vi "000 Data Edit Panel.vi"() -> (2 "OK?":bool)   [LabVIEW 2020]
panel:
  in  "Cancle":bool
  in  "OK":bool
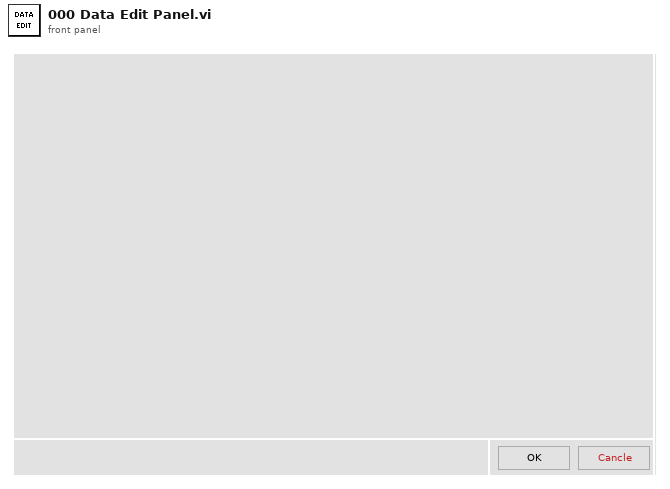
[diagram p1: front panel]
types:
  T1 = cluster{"UI":refnum<queue>, "UE":refnum<user-event>}
  T2 = cluster{"Queue":cluster{"UI":refnum<queue>, "UE":refnum<user-event>}, "OK?":bool}
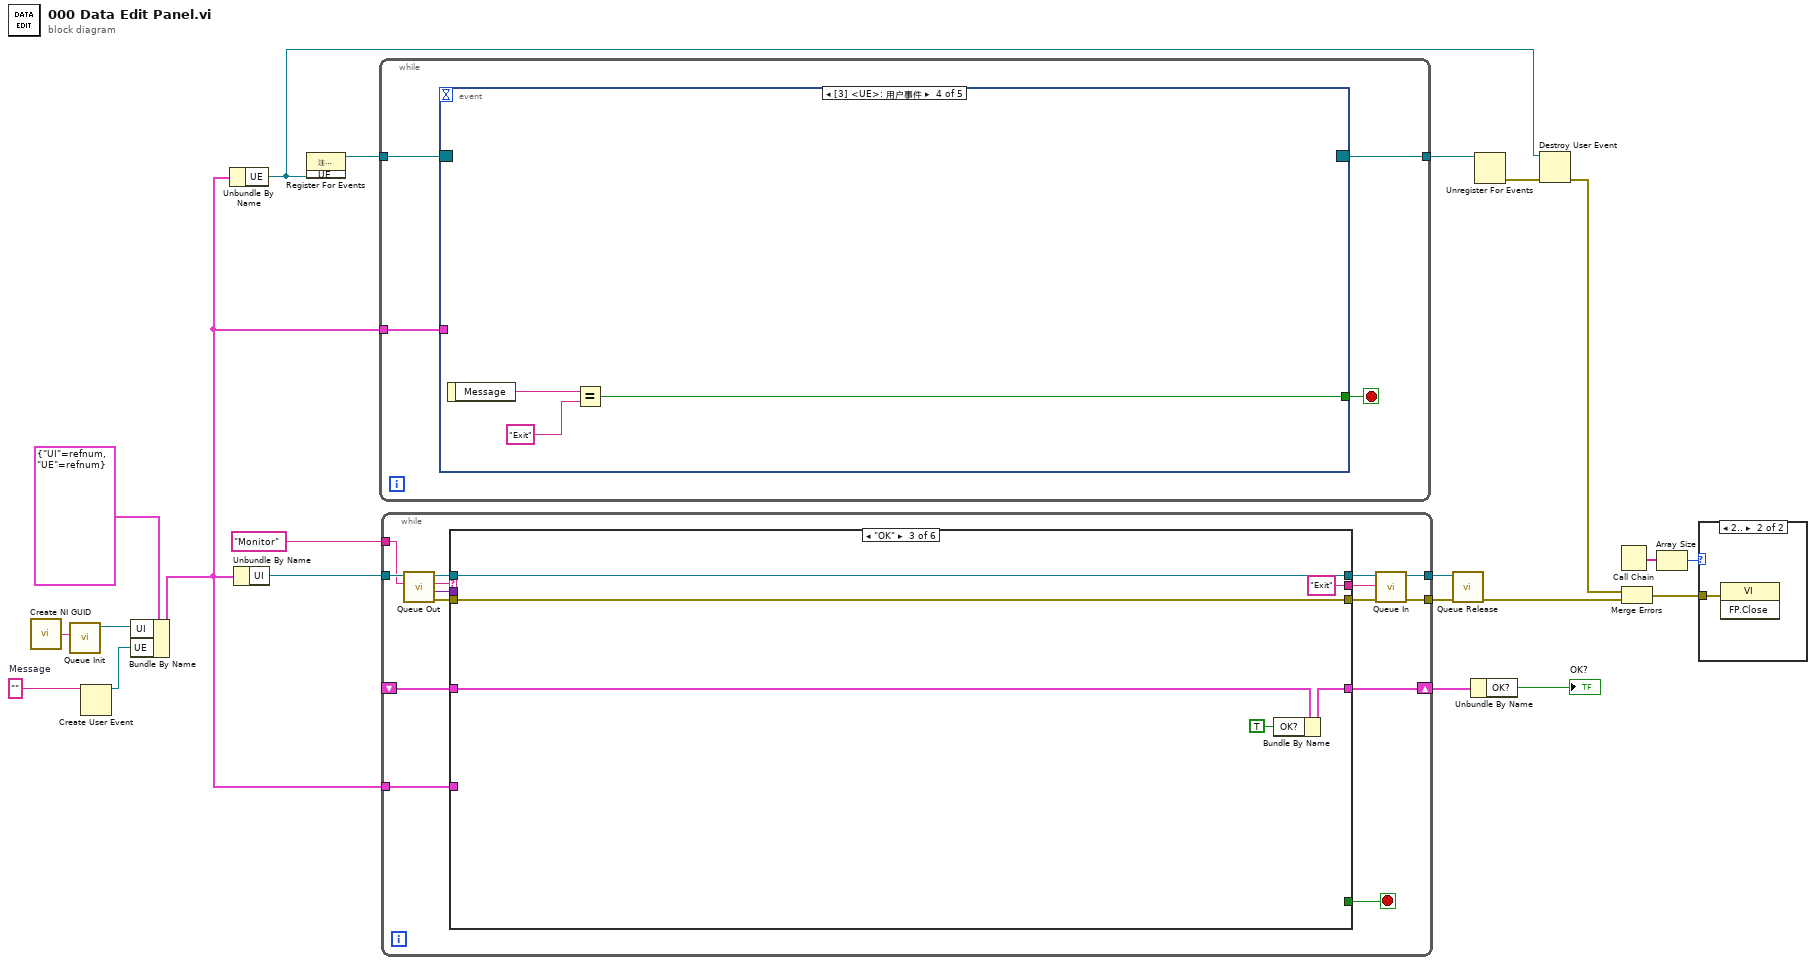
[diagram p0: block diagram]
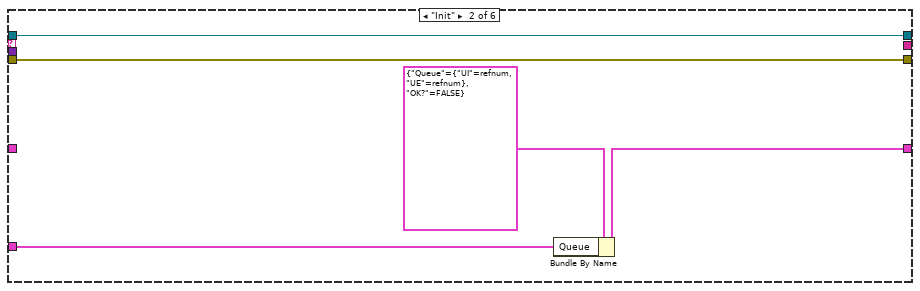
[diagram p4: hidden frame]
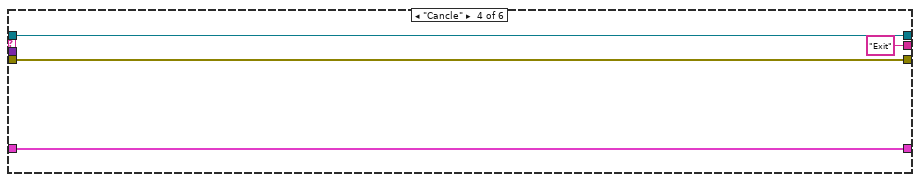
[diagram p5: hidden frame]
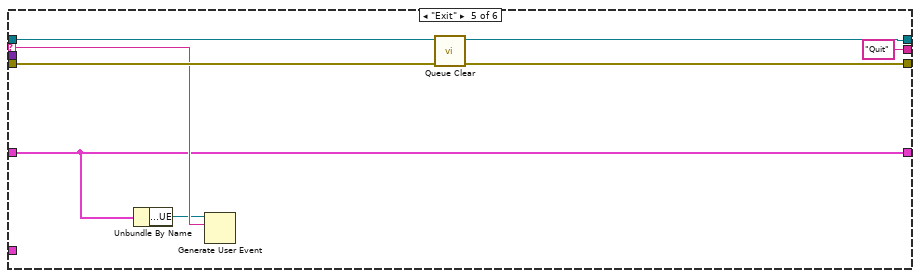
[diagram p6: hidden frame]
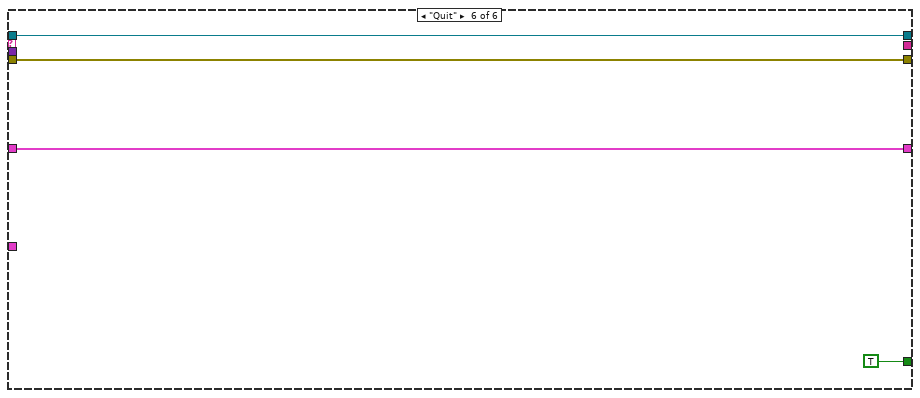
[diagram p7: hidden frame]
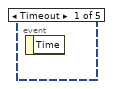
[diagram p8: hidden frame]
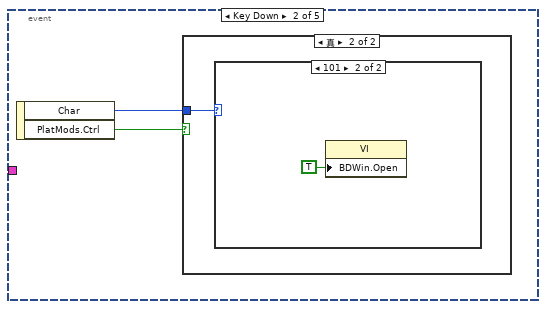
[diagram p9: hidden frame]
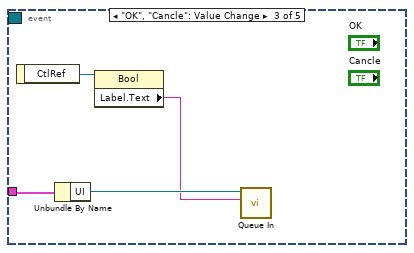
[diagram p12: hidden frame]
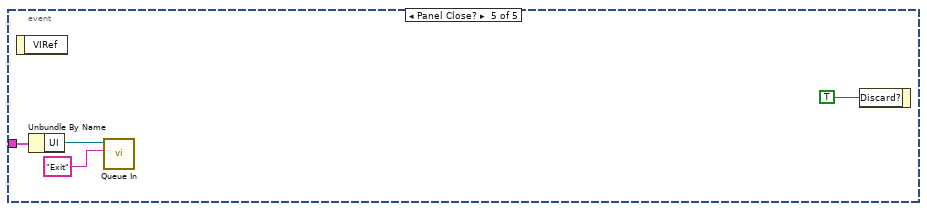
[diagram p13: hidden frame]
diagram:
  w10 = ""  # Message
  n1 = call <vilib>:"Create NI GUID.vi"() -> ("NI GUID"=w8:string)
  n2 = call "Queue Init.vi"("Queue Name"=w8) -> ("Queue Out"=w7:refnum<queue>)  [unwired: 8 in, 2 out]
  n3 = Create User Event(user event datatype=w10) -> (user event=w6:refnum<user-event>)  [unwired: 1 in, 1 out]
  n4 = Bundle By Name(cluster=T1 {"UI"=refnum, "UE"=refnum} ("Queue Ref Out"), "UI"=w7, "UE"=w6) -> (w5:T1)
  n5 = Unbundle By Name(w5) -> ("UE"=w4:refnum<user-event>)
  n6 = Unbundle By Name(w5) -> ("UI"=w16:refnum<queue>)
  n7 = register-events(w4) -> (reference out=w11:refnum<event-registration>)  [unwired: 2 in, 1 out]
  n8 = while {
    tunnel: w11 -> [w25]
    tunnel: [w23] -> w12
    tunnel: w5 -> [w22]
    stop <- w24 stop-if-true
    n9 = event shown="[3] <UE>: 用户事件" {
      selector: w25 -> [_ _ _ _ _]
      dyn-events: [_ _ _ _ _] -> w23
      timeout: _ -> [_ _ _ _ _]
      tunnel: [_ _ _ w34 _] -> w24
      tunnel: w22 -> [_ _ w33 _ w39]
      event Timeout {
        n10 = event-data() -> ()  [unwired: 1 in, 1 out]
      }
      event Key Down {
        n11 = event-data() -> ("Char"=w27:i16, "PlatMods.Ctrl"=w26:bool)  [unwired: 1 in]
        n12 = case shown="真" w26 {
          tunnel: w27 -> [_ w28]
          frame False {
          }
          frame True {
            n13 = case shown="101" w28 {
              frame 0, Default {
              }
              frame 101 {
                n14 = property class="VI"("BDWin.Open"=TRUE ("程序框图窗口:打开")) -> ()  [unwired: 2 in, 2 out]
              }
            }
          }
        }
      }
      event "OK", "Cancle": Value Change {
        n15 = event-data() -> ("CtlRef"=w31:refnum<vi>)  [unwired: 1 in]
        n16 = Unbundle By Name(w33) -> ("UI"=w32:refnum<queue>)
        n17 = property class="Bool"(reference=w31) -> ("Label.Text"=w30:string)  [unwired: 1 in, 2 out]
        n18 = call "Queue In.vi"("Message"=w30, "Queue In"=w32) -> ()  [unwired: 8 in, 2 out]
      }
      event User Event {
        n19 = event-data() -> ("Message"=w36:string)  [unwired: 1 in]
        n20 = Equal?(x=w36, y="Exit") -> (x = y?=w34:bool)
      }
      event Panel Close? {
        n21 = event-data() -> ()  [unwired: 1 in, 1 out]
        n22 = Unbundle By Name(w39) -> ("UI"=w38:refnum<queue>)
        n23 = call "Queue In.vi"("Message"="Exit", "Queue In"=w38) -> ()  [unwired: 8 in, 2 out]
        n24 = event-data("Discard?"=TRUE ("放弃？")) -> ()  [unwired: 1 in, 1 out]
      }
    }
  }
  n25 = while {
    tunnel: w16 -> [w51]
    tunnel: [w48] -> w14
    tunnel: [w47] -> w15
    tunnel: w5 -> [w44]
    shift-right: [w43] -> w3
    shift-left: _ -> [w42]
    tunnel: "Monitor" ("Monitor") -> [w41]
    stop <- w55 stop-if-true
    n26 = call "Queue Out.vi"("Monitor"=w41, "Queue In"=w51) -> ("error out"=w54:errorcluster, "Data"=w52:variant, "Message"=w53:string, "Queue Out"=w50:refnum<queue>)  [unwired: 5 in, 1 out]
    n27 = case shown="\"OK\"" w53 {
      selector: w53 -> [_ _ _ _ w76 _]
      tunnel: w50 -> [w58 w63 w69 w73 w80 w84]
      tunnel: w54 -> [w57 w62 w68 w72 w78 w85]
      tunnel: [w58 w63 w69 w73 w79 w84] -> w49
      tunnel: [w57 w62 w68 w72 w77 w85] -> w46
      tunnel: [_ _ "Exit" "Exit" "Quit" _] -> w45
      tunnel: [_ _ _ _ _ TRUE] -> w55
      tunnel: w52 -> [_ _ _ _ _ _]
      tunnel: w44 -> [_ w59 _ _ _ _]
      tunnel: [w56 w60 w66 w71 w74 w82] -> w43
      tunnel: w42 -> [w56 _ w67 w71 w74 w82]
      frame "eee", Default {
      }
      frame "Init" {
        n28 = Bundle By Name(cluster=T2 {"Queue"={"UI"=refnum, "UE"=refnum}, "OK?"=FALSE}, "Queue"=w59) -> (w60:T2)
      }
      frame "OK" {
        n29 = Bundle By Name(cluster=w67, "OK?"=TRUE) -> (w66:T2)
      }
      frame "Cancle" {
      }
      frame "Exit" {
        n30 = Unbundle By Name(w74) -> ("Queue.UE"=w75:refnum<user-event>)
        n31 = Generate User Event(user event=w75, event data cluster=w76) -> ()  [unwired: 2 in, 2 out]
        n32 = call "Queue Clear.vi"("error in (no error)"=w78, "Queue In"=w80) -> ("error out"=w77:errorcluster, "Queue Out"=w79:refnum<queue>)  [unwired: 8 in]
      }
      frame "Quit" {
      }
    }
    n33 = call "Queue In.vi"("error in (no error)"=w46, "Message"=w45, "Queue In"=w49) -> ("error out"=w47:errorcluster, "Queue Out"=w48:refnum<queue>)  [unwired: 7 in]
  }
  n34 = call "Queue Release.vi"("error in (no error)"=w15, "Queue In"=w14) -> ("error out"=w18:errorcluster)  [unwired: 9 in]
  n35 = Unbundle By Name(w3) -> ("OK?"=→"OK?":bool)
  n36 = Unregister For Events(event registration refnum=w12) -> (error out=w13:errorcluster)  [unwired: 1 in]
  n37 = Destroy User Event(user event=w4, error in=w13) -> (error out=w17:errorcluster)
  n38 = Call Chain() -> (call chain=w20:string[])
  n39 = Merge Errors(w17, w18) -> (w19:errorcluster)
  n40 = Array Size(array=w20) -> (size(s)=w21:i32)
  n41 = case shown="2.." w21 {
    tunnel: w19 -> [_ w86]
    frame 0, Default {
    }
    frame 2.. {
      n42 = invoke class="VI" method="FP.Close"(error in=w86) -> ()  [unwired: 2 in, 3 out]
    }
  }
